vi "Replicate.vi"(4 "Runner.lvclass":refnum<class "Runner.lvclass">, 6 "Direction":T1, 7 "Next Play":u32, 9 "YX Type":string, 11 "Maze 2.0.lvclass":refnum<class "SquareBattle.lvclass">) -> (1 "Success?":bool)   [LabVIEW 2014, in "SquareBattle.lvclass"]
uses:
  SquareBattle.lvclass
  Direction Enum.ctl
  Runner/Runner.lvclass
  Runner Cluster.ctl
  SquareBattle.lvclass/SquareBattle.ctl
panel:
  # "NOTICE - YOU MUST NOT REMOVE THIS NOTICE. PER THE FOLLOWING LICENSE, YOU MAY REPRODUCE THIS SOFTWARE PROVIDED YOU FOLLOW THE TERMS\nOF THE LICENSE.\n\n---BEGIN BSD LICENSE (http://opensource.org/licenses/BSD-2-Clause)---\nCopyright (c) 2015, Endigit, Inc. <robert@endigit.com>\nAll rights reserved.\n\nRedistribution and use in source and binary forms, with or without modification, are permitted provided that the following conditions are met:\n\n1. Redistributions of source code must retain the above copyright notice, this list of conditions and the following disclaimer.\n\n2. Redistributions in binary form must reproduce the above copyright notice, this list of conditions and the following disclaimer in the documentation and/or other \nmaterials provided with the distribution.\n\nTHIS SOFTWARE IS PROVIDED BY THE COPYRIGHT HOLDERS AND CONTRIBUTORS \"AS IS\" AND ANY EXPRESS OR IMPLIED WARRANTIES, INCLUDING, BUT NOT \nLIMITED TO, THE IMPLIED WARRANTIES OF MERCHANTABILITY AND FITNESS FOR A PARTICULAR PURPOSE ARE DISCLAIMED. IN NO EVENT SHALL THE COPYRIGHT \nHOLDER OR CONTRIBUTORS BE LIABLE FOR ANY DIRECT, INDIRECT, INCIDENTAL, SPECIAL, EXEMPLARY, OR CONSEQUENTIAL DAMAGES (INCLUDING, BUT NOT \nLIMITED TO, PROCUREMENT OF SUBSTITUTE GOODS OR SERVICES; LOSS OF USE, DATA, OR PROFITS; OR BUSINESS INTERRUPTION) HOWEVER CAUSED AND ON \nANY THEORY OF LIABILITY, WHETHER IN CONTRACT, STRICT LIABILITY, OR TORT (INCLUDING NEGLIGENCE OR OTHERWISE) ARISING IN ANY WAY OUT OF THE USE \nOF THIS SOFTWARE, EVEN IF ADVISED OF THE POSSIBILITY OF SUCH DAMAGE.\n---END BSD LICENSE---"
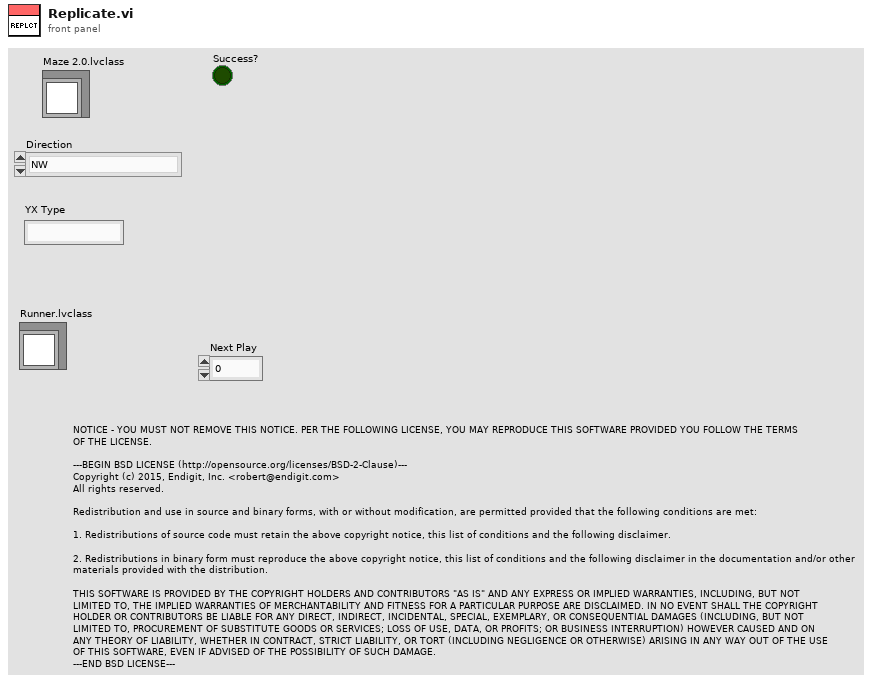
[diagram p1: front panel]
types:
  T1 = typedef "SquareBattle.lvclass/Direction Enum.ctl" = enum16{"NW", "N", "NE", "E", "SE", "S", "SW", "W"}
  T2 = typedef "SquareBattle.lvclass/Runner Cluster.ctl" = cluster{"Alive?":bool, "RunnerRef":refnum<data-value>, "TeamIdx":i32, "Player #":i32, "NextPlay":u32}
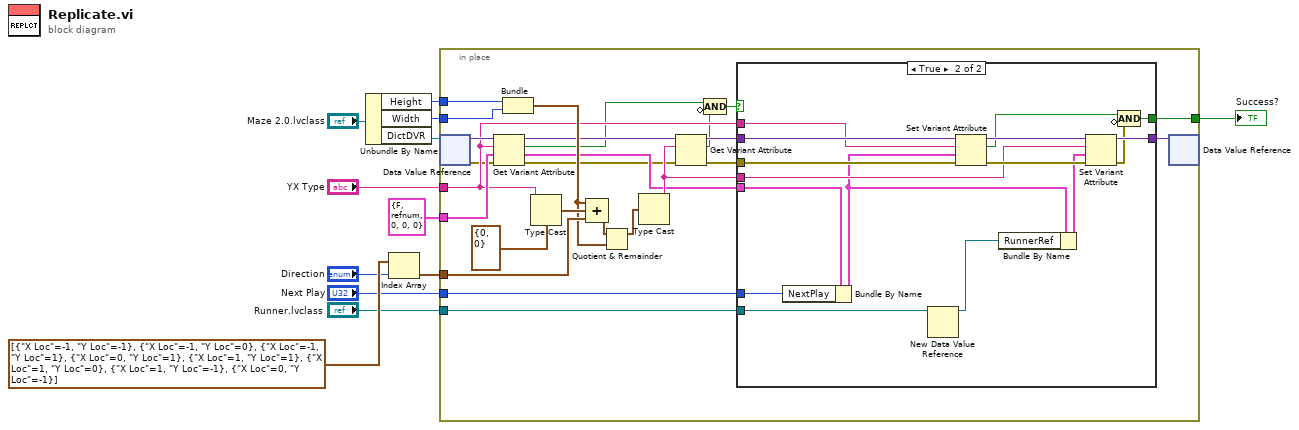
[diagram p0: block diagram]
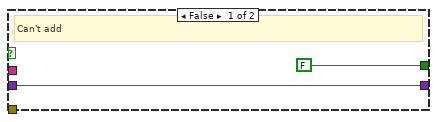
[diagram p2: hidden frame]
diagram:
  n1 = Unbundle By Name("Maze 2.0.lvclass") -> ("Height"=w5:i32, "Width"=w4:i32, "DictDVR"=w6:refnum<data-value>)
  n2 = Index Array(array=cluster{"X Loc":i32, "Y Loc":i32}[] [{"X Loc"=-1, "Y Loc"=-1}, {"X Loc"=-1, "Y Loc"=0}, {"X Loc"=-1, "Y Loc"=1}, {"X Loc"=0, "Y Loc"=1}, {"X Loc"=1, "Y Loc"=1}, {"X Loc"=1, "Y Loc"=0}, {"X Loc"=1, "Y Loc"=-1}, {"X Loc"=0, "Y Loc"=-1}], index="Direction") -> (element=w8:cluster{"X Loc":i32, "Y Loc":i32})
  n3 = in-place {
    in-place-border: "YX Type" -> [w19]
    in-place-border: T2 {"Alive?"=FALSE, "RunnerRef"=refnum, "TeamIdx"=0, "Player #"=0, "NextPlay"=0} ("Cluster") -> [w36]
    in-place-border: w8 -> [w31]
    in-place-border: w5 -> [w35]
    in-place-border: w4 -> [w34]
    in-place-border: [w24] -> w3
    in-place-border: "Next Play" -> [w18]
    in-place-border: "Runner.lvclass" -> [w13]
    n4 = in-place-dvr #1(w6) -> (w37:variant, w14:errorcluster)
    n5 = Get Variant Attribute(Variant=w37, name=w19, default value (empty Variant)=w36, error in=w14) -> (duplicate Variant=w27:variant, found=w17:bool, value=w22:T2, error out=w20:errorcluster)
    n6 = Bundle("Height"=w35, "Width"=w34) -> (w29:cluster{"Height":i32, "Width":i32})  [unwired: 1 in]
    n7 = Type Cast(type=cluster{"Y":i32, "X":i32} {"Y"=0, "X"=0}, x=w19) -> (*(type *) &x=w30:cluster{"Y":i32, "X":i32})
    n8 = Compound Arithmetic op=ADD(w29, w30, w31) -> (w33:cluster{i32, i32})
    n9 = Quotient & Remainder(x=w33, y=w29) -> (x-y*floor(x/y)=w28:cluster{i32, i32})  [unwired: 1 out]
    n10 = Type Cast(x=w28) -> (*(type *) &x=w23:string)  [unwired: 1 in]
    n11 = Get Variant Attribute(Variant=w27, name=w23, error in=w20) -> (duplicate Variant=w26:variant, found=w16:bool, error out=w21:errorcluster)  [unwired: 1 in, 1 out]
    n12 = Compound Arithmetic op=AND(w17, invert w16) -> (w15:bool)
    n13 = case shown="True" w15 {
      tunnel: w26 -> [w39 w55]
      tunnel: [w39 w48] -> w25
      tunnel: [FALSE w53] -> w24
      tunnel: w23 -> [_ w44]
      tunnel: w22 -> [_ w51]
      tunnel: w21 -> [_ w54]
      tunnel: w19 -> [_ w50]
      tunnel: w18 -> [_ w52]
      tunnel: w13 -> [_ w40]
      frame False {
        # "Can't add"
      }
      frame True {
        n14 = Bundle By Name(cluster=w51, "NextPlay"=w52) -> (w43:T2)
        n15 = New Data Value Reference(data value=w40) -> (data value reference=w42:refnum<data-value>)  [unwired: 1 in, 1 out]
        n16 = Set Variant Attribute(Variant=w55, name=w50, value=w43, error in=w54) -> (Variant out=w49:variant, replaced=w45:bool, error out=w47:errorcluster)
        n17 = Bundle By Name(cluster=w43, "RunnerRef"=w42) -> (w41:T2)
        n18 = Set Variant Attribute(Variant=w49, name=w44, value=w41, error in=w47) -> (Variant out=w48:variant, error out=w46:errorcluster)  [unwired: 1 out]
        n19 = Compound Arithmetic op=AND(w45, invert w46) -> (w53:bool)
      }
    }
    n20 = in-place-dvr #1(w25) -> ()  [unwired: 2 out]
  }
  "Success?" <- w3
